vi "Sub_FastDcvWithRemoveReadings.vi"(0 "IO Address":string="GPIB0::22::INSTR", 1 "Sample Source":enum16{"Timer", "Immediate"}(ring)=enum."Immediate", 2 "Data Format":enum16{"ASCII", "Real"}(ring)=enum."Real", 5 "サンプリング間隔":dbl=0.01, 7 "サンプルデータ数":i32=4000 min=1 max=1000000 step=1, 9 "Voltage Range":T4(ring)=enum."10 V", 11 "Integraton Time\nFunction":T2(ring), 12 "Trigger Source":T3(ring), 13 "Trig Delay Auto":bool, 14 "Trigger Delay (0 sec)":dbl, 15 "Trigger Slope (1:Falling Edge)":enum16{"Rising Edge", "Falling Edge"}(ring)=enum."Falling Edge") -> (4 "Measurement Results":dbl[](array[numeric]) format="%1_9f", 6 "波形グラフ":T1(graph)={0, 0.01, "Output Data (Numbers Only)"=[]}, 8 "error out":errorcluster)   [LabVIEW 2017]
panel:
  out "待ち時間(秒）":dbl
  # "Fast DC Voltage Measurementl"
  # "This example shows how to set up the DMM for very fast DC measurements and how to\nread out a specific number of data points using the binary (Real) data format for\nfastest execution.  Selecting ASCII for the Data Format will result in slower data\ntransfers from memory because more bytes are used to represent each data point.\n\n2006.6.28 *OPC? 書き込みの後に、データサンプル時間の遅延を入れた　川島"
  # "seconds"
  # "GPIB0::22::INSTR"
  # "10ms: 0,01\n150ms: 0.15"
  # "10V"
  # "REAL 64bit"
  # "MIN 10"
  # "DC VOLTS"
  # "IMMEDIATE"
  # "OFF"
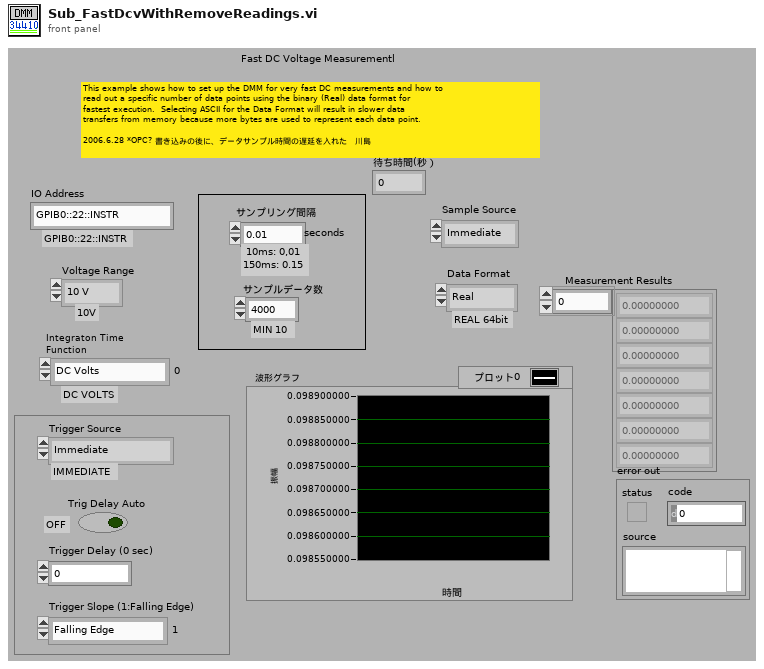
[diagram p1: front panel]
types:
  T1 = cluster{i32, dbl, "Output Data (Numbers Only)":dbl[]}
  T2 = enum16{"DC Volts", "2-Wire Resistance", "4-Wire Resistance", "DC Current", "Temperature"}
  T3 = enum16{"Immediate", "External", "Bus", "Internal (34411 Only)"}
  T4 = enum16{"100 mV", "1 V", "10 V", "100 V", "1000 V", "Auto", "Minimum", "Maximum"}
  T5 = cluster{i32, "サンプリング間隔":dbl, "Output Data (Numbers Only)":dbl[]}
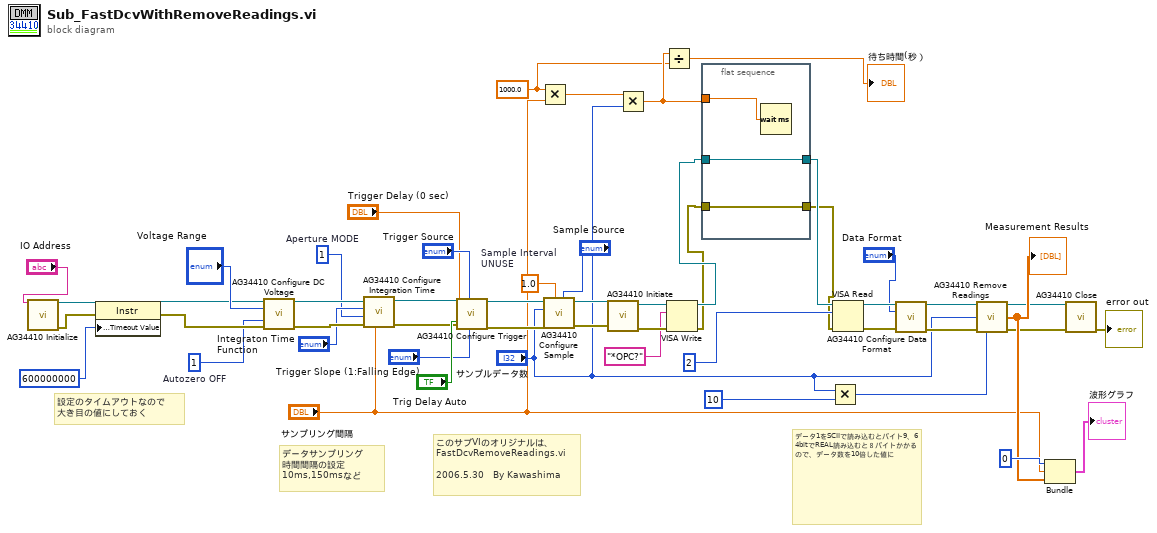
[diagram p0: block diagram]
diagram:
  w4 = 1000.0 ("x")
  w39 = 1.0  # Sample Interval UNUSE
  w16 = 1  # Autozero OFF
  w17 = 1  # Aperture MODE
  # "このサブVIのオリジナルは、\nFastDcvRemoveReadings.vi\n\n2006.5.30　By Kawashima"
  # "設定のタイムアウトなので\n大き目の値にしておく"
  # "データサンプリング\n時間間隔の設定\n10ms,150msなど"
  # "データ1をSCIIで読み込むとバイト9、64bitでREAL読み込むと８バイトかかるので、データ数を10倍した値に"
  n1 = call "AG34410 Initialize.vi"("VISA resource name"="IO Address") -> ("VISA resource name out"=w50:refnum<visa-resource-name>, "error out"=w51:errorcluster)  [unwired: 13 in]
  n2 = property class="Instr"(reference=w50, error in=w51, "General Settings:Timeout Value"=600000000) -> (reference out=w31:refnum<visa-resource-name>, error out=w49:errorcluster)
  n3 = call "AG34410 Configure DC Voltage.vi"("VISA resource name"=w31, "Range (5:Auto)"="Voltage Range", "Autozero (0:ON)"=w16, "error in (no error)"=w49) -> ("VISA resource name out"=w30:refnum<visa-resource-name>, "error out"=w28:errorcluster)  [unwired: 10 in]
  n4 = call "AG34410 Configure Integration Time.vi"("Aperture Value(100uS)"="サンプリング間隔", "error in (no error)"=w28, "Mode(0:NPLC)"=w17, "Function (0:DC Volts)"="Integraton Time\nFunction", "VISA resource name"=w30) -> ("error out"=w27:errorcluster, "VISA resource name out"=w29:refnum<visa-resource-name>)  [unwired: 5 in]
  n5 = call "AG34410 Configure Trigger.vi"("VISA resource name"=w29, "Trigger Delay (0 sec)"="Trigger Delay (0 sec)", "Trigger Delay Auto (T:On)"="Trig Delay Auto", "error in (no error)"=w27, "Trigger Source (0:Immediate)"="Trigger Source", "Trigger Slope (1:Falling Edge)"="Trigger Slope (1:Falling Edge)") -> ("VISA resource name out"=w37:refnum<visa-resource-name>, "error out"=w36:errorcluster)  [unwired: 12 in]
  n6 = Multiply(x=w4, y="サンプリング間隔") -> (x*y=w6:dbl)
  n7 = call "AG34410 Configure Sample.vi"("Sample Source (1:Immediate)"="Sample Source", "Sample Interval (1 sec)"=w39, "error in (no error)"=w36, "Sample Count (1)"="サンプルデータ数", "VISA resource name"=w37) -> ("error out"=w41:errorcluster, "VISA resource name out"=w40:refnum<visa-resource-name>)  [unwired: 5 in]
  n8 = call "AG34410 Initiate.vi"("VISA resource name"=w40, "error in (no error)"=w41) -> ("VISA resource name out"=w48:refnum<visa-resource-name>, "error out"=w47:errorcluster)  [unwired: 12 in]
  n9 = Multiply(x=w6, y="サンプルデータ数") -> (x*y=w5:dbl)
  n10 = Divide(x=w5, y=w4) -> (x/y=→"待ち時間(秒）":dbl)
  n11 = VISA Write(VISA resource name=w48, write buffer="*OPC?", error in (no error)=w47) -> (VISA resource name out=w12:refnum<visa-resource-name>, error out=w10:errorcluster)  [unwired: 1 out]
  n12 = flat-sequence {
    tunnel: w12 -> [w54]
    tunnel: [w54] -> w11
    tunnel: w10 -> [w53]
    tunnel: [w53] -> w9
    tunnel: w5 -> [w52]
    frame #0 {
      n13 = Wait (ms)(milliseconds to wait=w52) -> ()  [unwired: 1 out]
    }
  }
  n14 = Multiply(x="サンプルデータ数", y=10) -> (x*y=w18:i32)
  n15 = VISA Read(VISA resource name=w11, byte count=2, error in (no error)=w9) -> (VISA resource name out=w44:refnum<visa-resource-name>, error out=w43:errorcluster)  [unwired: 2 out]
  n16 = call "AG34410 Configure Data Format.vi"("VISA resource name"=w44, "Data Format (0:ASCII)"="Data Format", "error in (no error)"=w43) -> ("VISA resource name out"=w25:refnum<visa-resource-name>, "error out"=w24:errorcluster)  [unwired: 11 in]
  n17 = call "AG34410 Remove Readings.vi"("VISA resource name"=w25, "Num Readings (1)"="サンプルデータ数", "error in (no error)"=w24, "Byte Count (1024 bytes)"=w18) -> ("VISA resource name out"=w2:refnum<visa-resource-name>, "Output Data (Numbers Only)"=w22:dbl[], "error out"=w1:errorcluster)  [unwired: 9 in]
  "Measurement Results" <- w22
  n18 = Bundle(0, "サンプリング間隔"="サンプリング間隔", "Output Data (Numbers Only)"=w22) -> (→"波形グラフ":T5)  [unwired: 1 in]
  n19 = call "AG34410 Close.vi"("VISA resource name"=w2, "error in (no error)"=w1) -> ("error out"=→"error out":errorcluster)  [unwired: 13 in]
